vi "QueueError.vi"(7 "QueRef":refnum<queue>, 11 "Error In":errorcluster[](array[cluster])) -> (3 "Error Out":errorcluster[](array[cluster]))   [LabVIEW 2014, in "BusController.lvlib"]
uses:
  BusController.lvlib
  QueueType.ctl
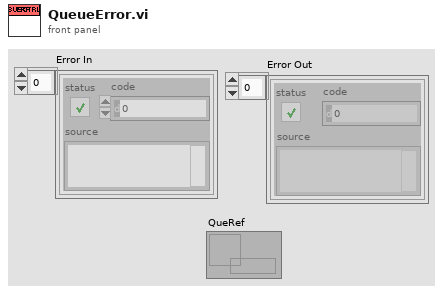
[diagram p1: front panel]
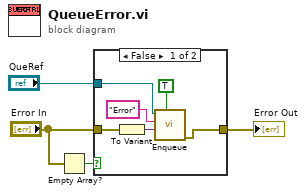
[diagram p0: block diagram]
diagram:
  n1 = Empty Array?(array="Error In") -> (empty?=w4:bool)
  n2 = case shown="False" w4 {
    tunnel: "Error In" -> [w10 _]
    tunnel: [w6 _] -> w2
    tunnel: "QueRef" -> [w5 _]
    frame False {
      n3 = To Variant(anything=w10) -> (Variant=w9:variant)
      n4 = call "Enqueue.vi"("Priority (f)"=TRUE, "Data"=w9, "Msg"="Error", "QueRef"=w5) -> ("Error Out"=w6:errorcluster[])  [unwired: 6 in, 1 out]
    }
    frame True {
    }
  }
  "Error Out" <- w2
